vi "Test_Insert_Image_ARGB_Mask_ARGB.vi"(8 "error in (no error)":errorcluster, 11 "Test Case In":refnum<class "Image.lvclass">) -> (0 "error out":errorcluster, 3 "Test Case Out":refnum<class "Image.lvclass">)   [LabVIEW 2020, in "g_ar_toolkit.test.lvlib" / "Image.lvclass"]
uses:
  Image.lvclass
  C:/Program Files (x86)/National Instruments/LabVIEW 2020/vi.lib/Astemes/LUnit/Test Case.lvclass
  g_ar_toolkit.image/Image Size (Fixed).ctl
  g_ar_toolkit.image/Image Point (Fixed).ctl
  g_ar_toolkit.image/ARGB Colour.ctl
  g_ar_toolkit.image/Line Type.ctl
  <vilib>/Astemes/LUnit/Test Case.lvclass/Test Case.ctl
  g_ar_toolkit.image/CreateEmptyImageARGB.vi
  g_ar_toolkit.image/DrawImageToPictureARGB.vi
  4993e8ee-a06a-463a-9684-69129f64d5ce.vi
  g_ar_toolkit.image/CreateEmptyImageARGB.vi/3321fa97-f432-4e1e-8db9-a0df79aed21b.vi
  g_ar_toolkit.image/DrawCircleOnImageARGB.vi/8336a1cf-e433-4bea-8080-376bdb783d4e.vi
  g_ar_toolkit.image/InsertImageARGBMaskARGB.vi/5e3288c8-ee88-4cfe-89cf-31ceca475f5a.vi
  g_ar_toolkit.image/DrawImageToPictureARGB.vi/8cd07b1b-062e-4fe4-9e87-2eb3dc89fe0e.vi
  <vilib>/Astemes/LUnit/Append Pass Result.vi
  <vilib>/Astemes/LUnit/Append Fail Result.vi
  <vilib>/Astemes/LUnit/Describe Comparison.vi
  <vilib>/Astemes/LUnit/Compare Variants.vi
  <vilib>/Astemes/LUnit/Variant to string.vi
  g_ar_toolkit.image/ARGBColourToU32.vi
  <vilib>/Utility/error.llb/Error Cluster From Error Code.vi
  <vilib>/Utility/Data Type/Get Type Information.vi
  <vilib>/Utility/LVClass/Get LV Class Name.vi
  Image.lvclass/Image.ctl
  g_ar_toolkit.image/g_ar_toolkit.image.lvlib
panel:
  out "Picture":picture
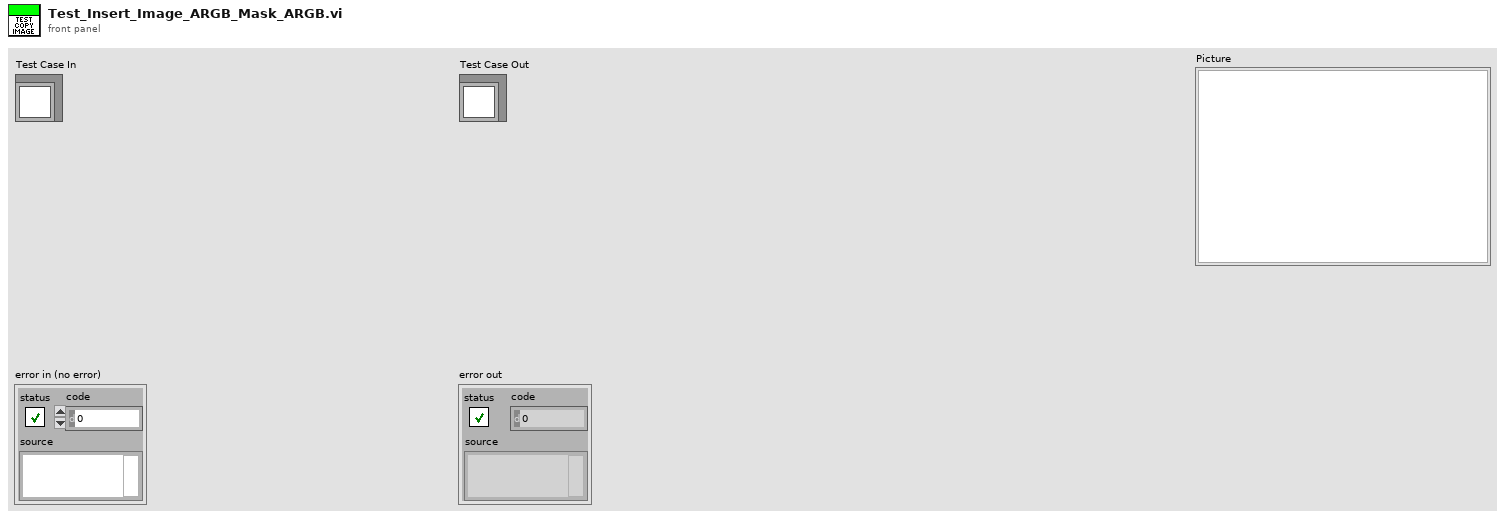
[diagram p1: front panel]
types:
  T1 = typedef "g_ar_toolkit.image.lvlib/Line Type.ctl" = enum8{"FILLED", "LINE_4", "LINE_8", "LINE_AA"}
  T2 = typedef "g_ar_toolkit.image.lvlib/ARGB Colour.ctl" = cluster{"Alpha":u8, "RGB":u32}
  T3 = typedef "g_ar_toolkit.image.lvlib/Image Point (Fixed).ctl" = cluster{"x":i32, "y":i32}
  T4 = typedef "g_ar_toolkit.image.lvlib/Image Size (Fixed).ctl" = cluster{"Width":u16, "Height":u16}
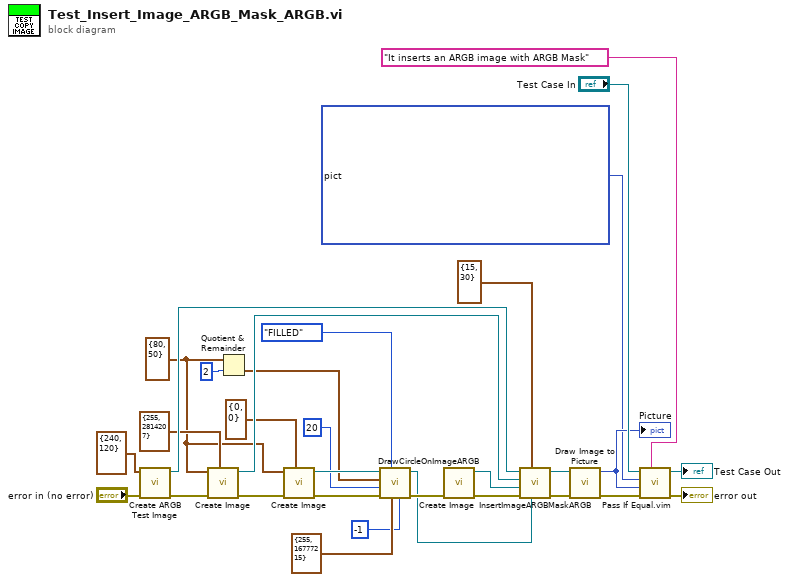
[diagram p0: block diagram]
diagram:
  w11 = T4 {"Width"=80, "Height"=50} ("Preallocated Image Size")
  n1 = call "Create ARGB Test Image.vi"("error in (no error)"="error in (no error)", "Preallocated Image Size"=T4 {"Width"=240, "Height"=120} ("Preallocated Image Size (Default - 0,0)")) -> ("error out"=w20:errorcluster, "Data Value Reference out"=w25:refnum<data-value>)  [unwired: 7 in, 1 out]
  n2 = call-poly "Create Image.vi"("Colour (Default: Black)"=T2 {"Alpha"=255, "RGB"=2814207}, "error in (no error)"=w20, "Preallocated Image Size (Default: 0,0)"=w11) -> ("error out"=w17:errorcluster, "New ARGB Image"=w19:refnum<data-value>)  [unwired: 7 in]
  n3 = Quotient & Remainder(x=w11, y=u16 2) -> (floor(x/y)=w9:T4)  [unwired: 1 out]
  n4 = call-poly "Create Image.vi"("Colour (Default: Black)"=T2 {"Alpha"=0, "RGB"=0}, "error in (no error)"=w17, "Preallocated Image Size (Default: 0,0)"=w11) -> ("error out"=w16:errorcluster, "New ARGB Image"=w15:refnum<data-value>)  [unwired: 7 in]
  n5 = call "DrawCircleOnImageARGB.vi"("Thickness (Default: 1)"=-1, "ARGB Colour"=T2 {"Alpha"=255, "RGB"=16777215}, "OpenCV Line Type (Default LINE_8)"=Line_Type."FILLED", "error in (no error)"=w16, "Radius"=u16 20, "Centre"=w9, "ARGB Image"=w15) -> ("error out"=w14:errorcluster, "ARGB Image (Duplicate)"=w13:refnum<data-value>)  [unwired: 3 in]
  n6 = call-poly "Create Image.vi"("error in (no error)"=w14) -> ("error out"=w27:errorcluster, "New ARGB Image"=w22:refnum<data-value>)  [unwired: 9 in]
  n7 = call "InsertImageARGBMaskARGB.vi"("ARGB Image Mask"=w13, "Offset (Default: 0,0)"=T3 {"x"=15, "y"=30}, "error in (no error)"=w27, "ARGB Image Destination"=w22, "ARGB Image Child"=w19, "ARGB Image Parent"=w25) -> ("error out"=w4:errorcluster, "ARGB Image Destination (duplicate)"=w21:refnum<data-value>)  [unwired: 4 in]
  n8 = call-poly "Draw Image to Picture.vi"("error in (no error)"=w4, "ARGB Image Source"=w21) -> ("error out"=w3:errorcluster, "Picture"=w2:picture)  [unwired: 8 in]
  "Picture" <- w2
  n9 = call "Pass If Equal.vim"("Description"="It inserts an ARGB image with ARGB Mask", "error in (no error)"=w3, "Actual"=w2, "Expected"=picture bytes[86430] ("Picture"), "LUnit Test Case In"="Test Case In") -> ("error out"=→"error out":errorcluster, "LUnit Test Case Out"=→"Test Case Out":refnum<class "Image.lvclass">)  [unwired: 5 in]
